vi "TL_read_setpoint.vi"(2 "setpoint #":i32, 3 "TL array":dbl[][](array[numeric])) -> (0 "QPD setpoint":cluster{"X":dbl, "Y":dbl, "intensity":dbl})   [LabVIEW 2015]
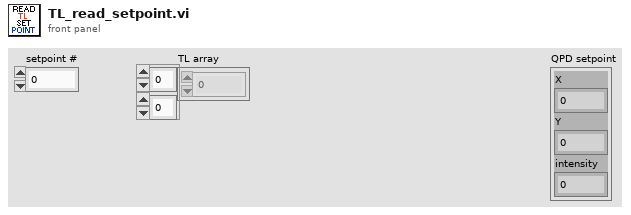
[diagram p1: front panel]
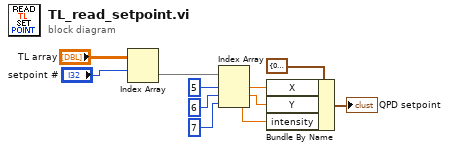
[diagram p0: block diagram]
diagram:
  n1 = Index Array(array="TL array", index (row)="setpoint #") -> (element=w1:dbl[])  [unwired: 1 in]
  n2 = Index Array(array=w1, index #1=5 ("index"), index #2=6 ("index"), index #3=7 ("index")) -> (element #1=w9:dbl, element #2=w10:dbl, element #3=w11:dbl)
  n3 = Bundle By Name(cluster=cluster{"X":dbl, "Y":dbl, "intensity":dbl} {"X"=0.0, "Y"=0.0, "intensity"=0.0} ("QPD ref"), "X"=w9, "Y"=w10, "intensity"=w11) -> (→"QPD setpoint":cluster{"X":dbl, "Y":dbl, "intensity":dbl})
